vi "Log.vi"(10 "Log Packet":T1, 11 "Buffered Log Sink in":refnum<class "Buffered String Log Sink.lvclass">) -> (0 "error out":errorcluster, 3 "Buffered Log Sink out":refnum<class "Buffered String Log Sink.lvclass">)   [LabVIEW 2019, in "Buffered String Log Sink.lvclass"]
uses:
  Buffered String Log Sink.lvclass
  Composed Log/Types/Log Packet.ctl
  Composed Log/Types/Log Level.ctl
  Buffered String Log Sink.lvclass/Buffered String Log Sink.ctl
  String Log Sink/String Log Sink.lvclass
  Composed Log/Composed Log.lvlib
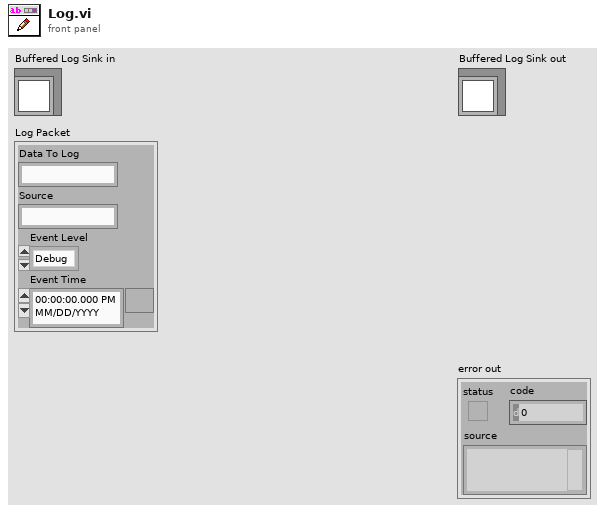
[diagram p1: front panel]
types:
  T1 = typedef "Composed Log.lvlib/Log Packet.ctl" = cluster{"Data To Log":string, "Source":string, "Event Level":T2, "Event Time":timestamp}
  T2 = typedef "Composed Log.lvlib/Log Level.ctl" = enum16{"Debug", "Info", "Warning", "Error", "Critical"}
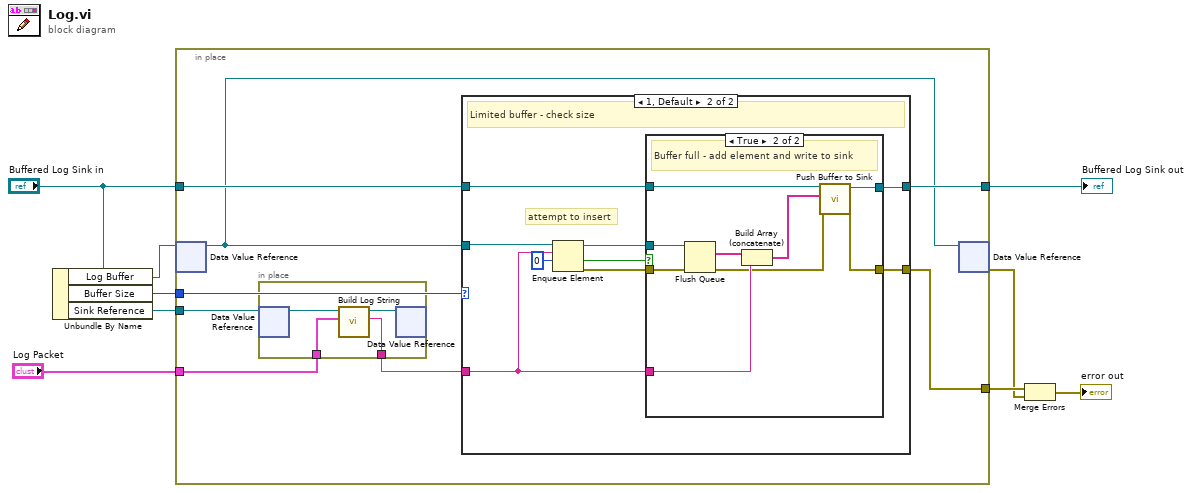
[diagram p0: block diagram]
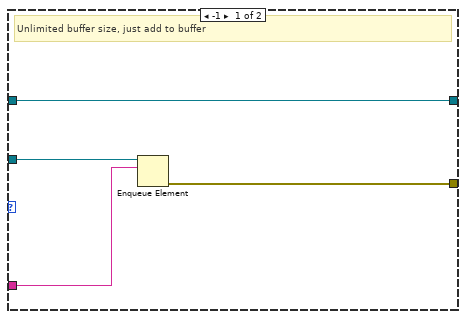
[diagram p2: hidden frame]
diagram:
  n1 = Unbundle By Name("Buffered Log Sink in") -> ("Log Buffer"=w4:refnum<data-value>, "Buffer Size"=w9:i32, "Sink Reference"=w1:refnum<data-value>)
  n2 = in-place {
    in-place-border: w9 -> [w17]
    in-place-border: "Log Packet" -> [w10]
    in-place-border: [w16] -> w7
    in-place-border: "Buffered Log Sink in" -> [w15]
    in-place-border: [w14] -> w5
    in-place-border: w1 -> [w12]
    n3 = in-place-dvr #1(w4) -> (w13:refnum<queue>)  [unwired: 1 out]
    n4 = in-place {
      in-place-border: w10 -> [w19]
      in-place-border: [w18] -> w11
      n5 = in-place-dvr #2(w12) -> (w21:refnum<class "String Log Sink.lvclass">)  [unwired: 1 out]
      n6 = call-dynamic "Build Log String.vi"("Log Packet"=w19, "String Log Sink in"=w21) -> ("Log Entry"=w18:string, "String Log Sink out"=w20:refnum<class "String Log Sink.lvclass">)  [unwired: 8 in]
      n7 = in-place-dvr #2(w20) -> ()  [unwired: 2 out]
    }
    n8 = case shown="1, Default" w17 {
      tunnel: w13 -> [w25 w31]
      tunnel: w11 -> [w24 w26]
      tunnel: [w23 w32] -> w16
      tunnel: w15 -> [w22 w34]
      tunnel: [w22 w33] -> w14
      frame -1 {
        # "Unlimited buffer size, just add to buffer"
        n9 = Enqueue Element(queue=w25, element=w24) -> (error out=w23:errorcluster)  [unwired: 2 in, 2 out]
      }
      frame 1, Default {
        # "attempt to insert"
        # "Limited buffer - check size"
        n10 = Enqueue Element(queue=w31, element=w26, timeout in ms (-1)=0) -> (queue out=w29:refnum<queue>, timed out?=w27:bool, error out=w30:errorcluster)  [unwired: 1 in]
        n11 = case shown="True" w27 {
          tunnel: w34 -> [w36 w41]
          tunnel: w30 -> [w35 w44]
          tunnel: w26 -> [_ w42]
          tunnel: w29 -> [_ w45]
          tunnel: [w36 w40] -> w33
          tunnel: [w35 w37] -> w32
          frame False {
            # "Nope - we're done here"
          }
          frame True {
            # "Buffer full - add element and write to sink"
            n12 = Flush Queue(queue=w45, error in (no error)=w44) -> (remaining elements=w43:string[], error out=w38:errorcluster)  [unwired: 1 out]
            n13 = Build Array (concatenate)(w43, w42) -> (w39:string[])
            n14 = call "Push Buffer to Sink.vi"("error in (no error)"=w38, "Strings to Log"=w39, "Buffered Log Sink in"=w41) -> ("error out"=w37:errorcluster, "Buffered Log Sink out"=w40:refnum<class "Buffered String Log Sink.lvclass">)  [unwired: 7 in]
          }
        }
      }
    }
    n15 = in-place-dvr #1(w13) -> (w2:errorcluster)  [unwired: 1 out]
  }
  "Buffered Log Sink out" <- w5
  n16 = Merge Errors(w7, w2) -> (→"error out":errorcluster)
